vi "Write TimeOut(s).vi"(8 "error in (no error)":errorcluster, 10 "TimeOut(s)":dbl, 11 "LT_UpgradeFlash in":refnum<class "LT_UpgradeFlash.lvclass">) -> (0 "error out":errorcluster, 3 "LT_UpgradeFlash out":refnum<class "LT_UpgradeFlash.lvclass">)   [LabVIEW 2017, in "LT_UpgradeFlash.lvclass"]
uses:
  LT_UpgradeFlash.lvclass
  LT_UpgradeFlash.lvclass/LT_UpgradeFlash.ctl
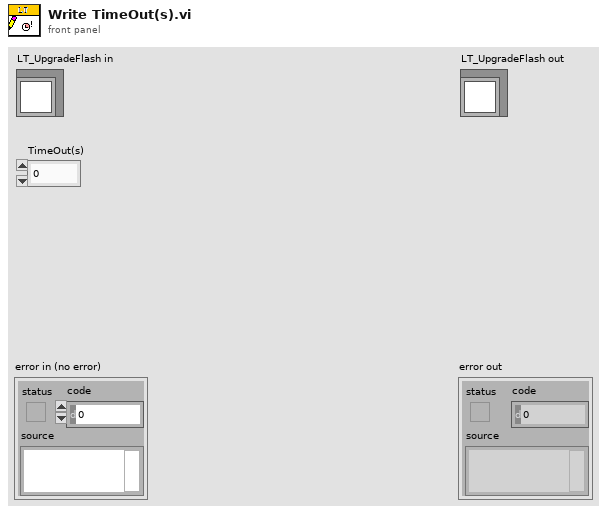
[diagram p1: front panel]
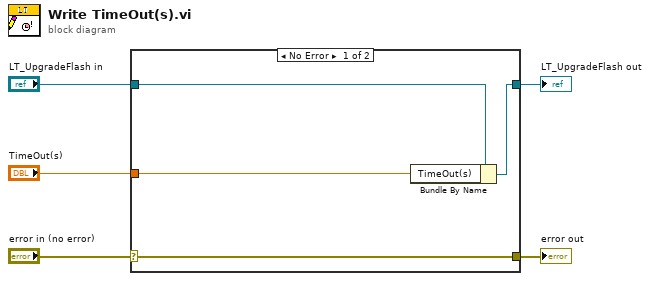
[diagram p0: block diagram]
diagram:
  n1 = case shown="No Error" "error in (no error)" {
    selector: "error in (no error)" -> [w9 w10]
    tunnel: [w9 w10] -> w4
    tunnel: [w7 w11] -> w2
    tunnel: "LT_UpgradeFlash in" -> [w8 w11]
    tunnel: "TimeOut(s)" -> [w6 _]
    frame No Error {
      n2 = Bundle By Name(cluster=w8, "TimeOut(s)"=w6) -> (w7:refnum<class "LT_UpgradeFlash.lvclass">)
    }
    frame Error {
    }
  }
  "error out" <- w4
  "LT_UpgradeFlash out" <- w2
